vi "Error Parser.vi"(8 "error in (no error)":errorcluster) -> (0 "Error out":errorcluster, 2 "Explanation":string, 3 "error?":bool)   [LabVIEW 2018]
doc: "This VI takes an error in and parses it to a string. It also shows a boolean in case there is an error."
uses:
  <vilib>/Utility/error.llb/DialogType.ctl
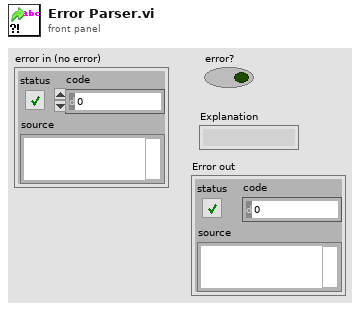
[diagram p1: front panel]
types:
  T1 = typedef "DialogType.ctl" = u16
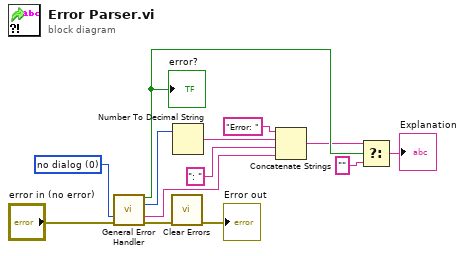
[diagram p0: block diagram]
diagram:
  w4 = T1 0 items=["no dialog", "OK message", "continue or stop message", "OK message + warnings", "continue/stop + warnings"] ("type of dialog (OK msg:1)")
  n1 = call <vilib>:"General Error Handler.vi"("type of dialog (OK msg:1)"=w4, "error in (no error)"="error in (no error)") -> ("error?"=w12:bool, "code out"=w5:i32, "message"=w9:string, "error out"=w2:errorcluster)  [unwired: 9 in, 1 out]
  "error?" <- w12
  n2 = call <vilib>:"Clear Errors.vi"("error in (no error)"=w2) -> ("error out"=→"Error out":errorcluster)  [unwired: 5 in, 1 out]
  n3 = Number To Decimal String(number=w5) -> (decimal integer string=w6:string)  [unwired: 1 in]
  n4 = Concatenate Strings("Error: " ("string"), w6, ": " ("string"), w9) -> (w11:string)
  n5 = Select(t=w11, s=w12, f="") -> (s? t:f=→"Explanation":string)
